vi "Get Time.vi"(8 "error in (no error)":errorcluster, 11 "ClockID":u8) -> (0 "error out":errorcluster, 3 "Time (ns)":u64, 5 "T0":u64)   [LabVIEW 2021, in "CIFClocks.lvlib"]
uses:
  CIFClocks.lvlib
  Typedef/Errors.ctl
  CIFCore/CIFCoreCommon/CIFCoreCommon.lvlib
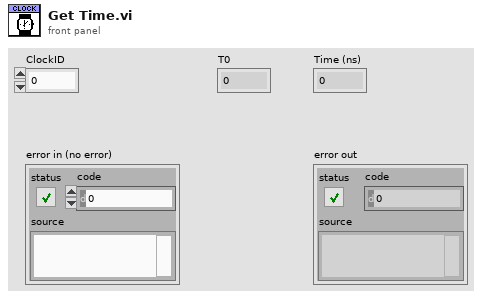
[diagram p1: front panel]
types:
  T1 = typedef "CIFCoreCommon.lvlib/Errors.ctl" = enum16{"Invalid Clock ID", "Long Sleep", "gRPC Server Not Found", "Config Parse", "Timestamp Wrap"}
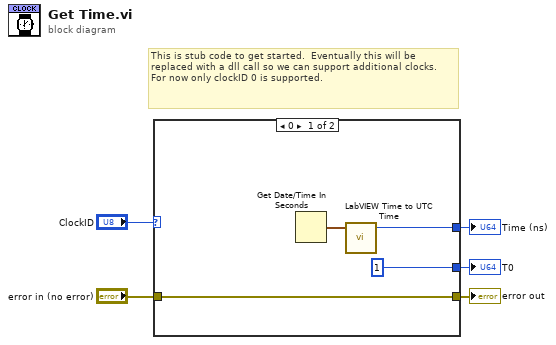
[diagram p0: block diagram]
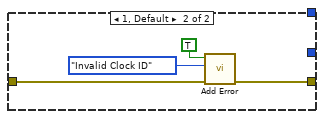
[diagram p2: hidden frame]
diagram:
  # "This is stub code to get started.  Eventually this will be replaced with a dll call so we can support additional clocks.  For now only clockID 0 is supported."
  n1 = case shown="0" "ClockID" {
    tunnel: [w7 _] -> w5
    tunnel: "error in (no error)" -> [w8 w13]
    tunnel: [w8 w12] -> w2
    tunnel: [u64 1 ("UTC Time (ns)") _] -> w1
    frame 0 {
      n2 = Get Date/Time In Seconds() -> (seconds since 1Jan1904=w9:timestamp)
      n3 = call "LabVIEW Time to UTC Time.vi"("LabVIEW Time (s)"=w9) -> ("UTC Time (ns)"=w7:u64)  [unwired: 4 in]
    }
    frame 1, Default {
      n4 = call "Add Error.vi"("error in (no error)"=w13, "Error"=Errors."Invalid Clock ID", "Insert Error"=TRUE) -> ("error out"=w12:errorcluster)  [unwired: 8 in]
    }
  }
  "error out" <- w2
  "Time (ns)" <- w5
  "T0" <- w1
